vi "Configure RF Power.vi"(8 "error in (no error)":errorcluster, 10 "power, W":u16, 11 "Comdel in":refnum<class "PL Comdel CX.lvclass">) -> (0 "error out":errorcluster, 3 "Comdel out":refnum<class "PL Comdel CX.lvclass">)   [LabVIEW 2015, in "PL Comdel CX.lvclass"]
doc: "Configures RF power value."
uses:
  PL Comdel CX.lvclass
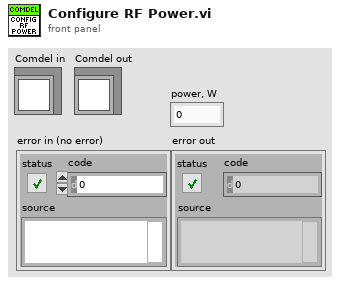
[diagram p1: front panel]
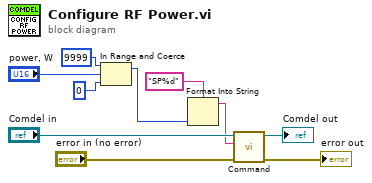
[diagram p0: block diagram]
diagram:
  n1 = In Range and Coerce(upper limit=u16 9999, x="power, W", lower limit=u16 0) -> (coerced(x)=w2:u16)  [unwired: 1 out]
  n2 = Format Into String(format string="SP%d", w2) -> (resulting string=w4:string)  [unwired: 2 in, 1 out]
  n3 = call "Command.vi"("error in (no error)"="error in (no error)", "command"=w4, "Comdel in"="Comdel in") -> ("error out"=→"error out":errorcluster, "Comdel out"=→"Comdel out":refnum<class "PL Comdel CX.lvclass">)  [unwired: 6 in, 1 out]
